vi "Read Compatible Hardware Types.vi"(8 "error in (no error)":errorcluster, 11 "Resistance in":refnum<class "Resistance.lvclass">) -> (0 "error out":errorcluster, 2 "Compatible Hardware Types":string[](array[string]), 3 "Resistance out":refnum<class "Resistance.lvclass">)   [LabVIEW 2013, in "Resistance.lvlib" / "Resistance.lvclass"]
uses:
  Resistance.lvclass
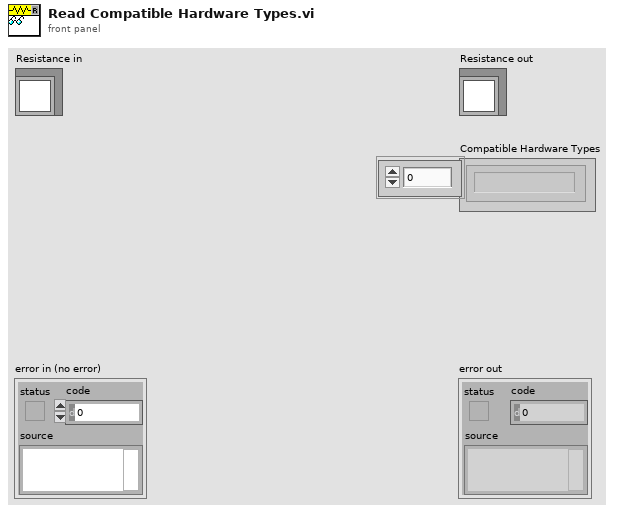
[diagram p1: front panel]
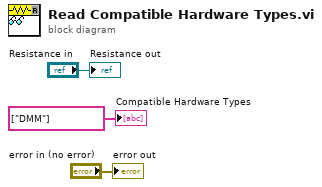
[diagram p0: block diagram]
diagram:
  "error out" <- "error in (no error)"
  "Resistance out" <- "Resistance in"
  "Compatible Hardware Types" <- string[] ["DMM"] ("Compatible Hardware Types")
